vi "Process Write.vi"(8 "error in (no error)":errorcluster, 10 "gRPCid":T1, 11 "Data Server":refnum<class "Data Server.lvclass">) -> (0 "error out":errorcluster)   [LabVIEW 2020, in "Veristandgrpc_server.lvlib" / "veristand-grpc.lvclass"]
uses:
  veristand-grpc.lvclass
  Data/Data Server.lvclass
  <vilib>/gRPC/LabVIEW gRPC Library/Shared/grpcId.ctl
  RPC Messages/veristand_Reponse.ctl
  Data/Data Server.lvclass/Data Server.ctl
  Veristandgrpc_server.lvlib
  <vilib>/gRPC/LabVIEW gRPC Library/grpc-lvsupport-release.lvlib
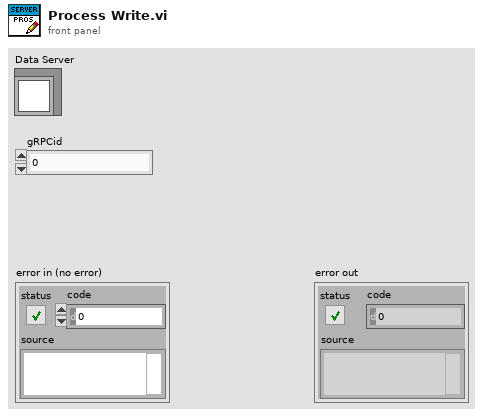
[diagram p1: front panel]
types:
  T1 = typedef "grpc-lvsupport-release.lvlib/grpcId.ctl" = u64
  T2 = typedef "Veristandgrpc_server.lvlib/veristand_Reponse.ctl" = cluster{"status":string, "data":string}
  T3 = typedef "Veristandgrpc_server.lvlib/veristand_Request.ctl" = cluster{"server":string, "channel":string, "data":string}
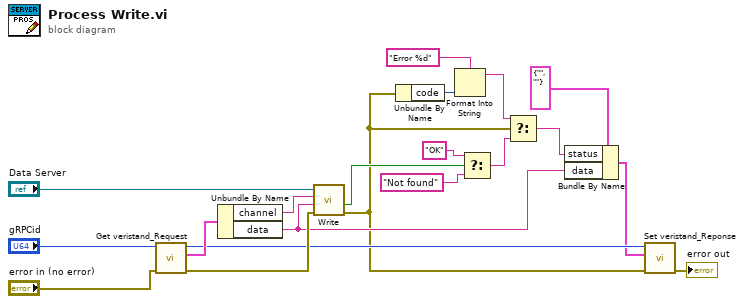
[diagram p0: block diagram]
diagram:
  n1 = call "Get veristand_Request.vi"("error in (no error)"="error in (no error)", "gRPCid"="gRPCid") -> ("error out"=w15:errorcluster, "package_templatemessage"=w18:T3, "gRPCid out"=w4:T1)  [unwired: 7 in]
  n2 = Unbundle By Name(w18) -> ("channel"=w16:string, "data"=w5:string)
  n3 = call "Write.vi"("error in (no error)"=w15, "New Data"=w5, "Channel Name"=w16, "Data in"="Data Server") -> ("error out"=w3:errorcluster, "Found"=w6:bool)  [unwired: 5 in, 1 out]
  n4 = Unbundle By Name(w3) -> ("code"=w12:i32)
  n5 = Format Into String(format string="Error %d", w12) -> (resulting string=w13:string)  [unwired: 2 in, 1 out]
  n6 = Select(t="OK" ("data"), s=w6, f="Not found" ("data")) -> (s? t:f=w8:string)
  n7 = Select(t=w13, s=w3, f=w8) -> (s? t:f=w14:string)
  n8 = Bundle By Name(cluster=T2 {"status"="", "data"=""} ("veristand_Reponse"), "status"=w14, "data"=w5) -> (w2:T2)
  n9 = call "Set veristand_Reponse.vi"("error in (no error)"=w3, "package_templatemessage"=w2, "gRPCid"=w4) -> ("error out"=→"error out":errorcluster)  [unwired: 8 in]
